vi "Passing Command Line Parameters.vi"() -> ()   [LabVIEW 2023]
doc: "This example shows how to use the Application:Command Line Arguments property to retrieve parameters that were returned when the LabVIEW executable was called from the command line.\n\nUse the following syntax in the Command Line to launch this VI:\n\n\"<full path to LabVIEW directory>\\labview.exe\" \"<full path to LabVIEW directory>\\examples\\Application Control\\VI Server\\Passing Command Line Parameters\\Command Line Target.vi\" This VI is set to run when opened.\n\nAfter the VI name, enter two hyphens (--) surrounded by spaces before the user-defined arguments. The arguments will be displayed in the front panel indicators. The correct syntax for arguments that can be passed is:\n\n/number:\n/boolean:\n/string:\nAfter (:) enter the appropriate value. If you enter more than one argument, they need to be separated with a space."
panel:
  out "Command Line String":string
  in  "String":string
  in  "Boolean":bool
  in  "Numeric":dbl
  # "Overview: Demonstrates how to call a VI, and pass parameters to the VI, through the command line.\nInstructions:\n1. Specify desired values for Numeric, Boolean and String.\n2. Run the VI.\n3. Highlight the text in the Command Line String indicator and select Edit > Copy to copy the text to the clipboard.\n4. Exit LabVIEW.\n5. Paste the string into a command line window and run the command. (To do this on Windows, press Window-R, type 'cmd', press Enter, right-click in the command window and select Paste, then press Enter.)"
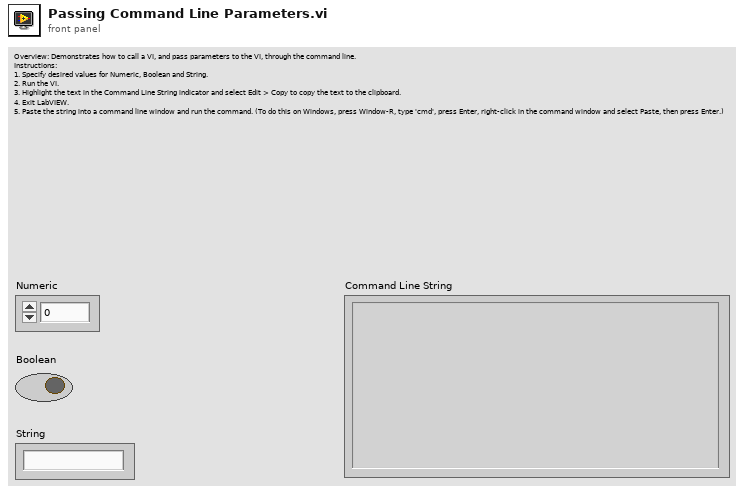
[diagram p1: front panel]
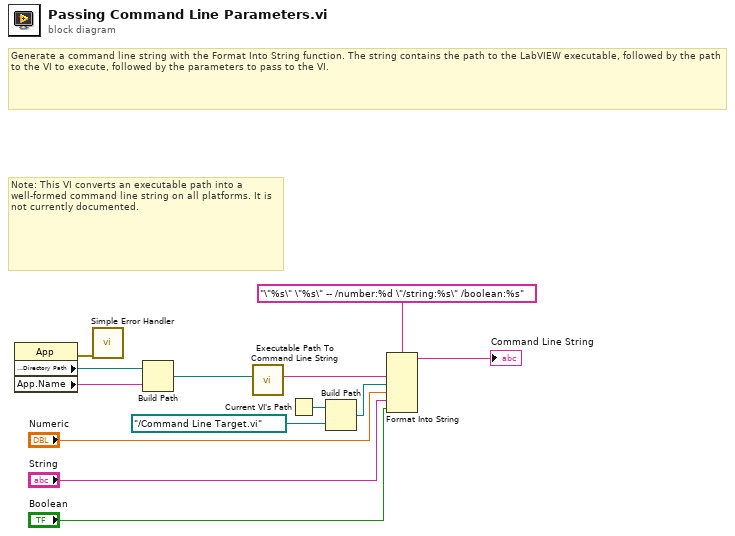
[diagram p0: block diagram]
diagram:
  # "Note: This VI converts an executable path into a well-formed command line string on all platforms. It is not currently documented."
  # "Generate a command line string with the Format Into String function. The string contains the path to the LabVIEW executable, followed by the path to the VI to execute, followed by the parameters to pass to the VI."
  n1 = property class="App"() -> (error out=w11:errorcluster, "Application:Directory Path"=w10:path, "App.Name"=w9:string)  [unwired: 2 in, 1 out]
  n2 = call <vilib>:"Simple Error Handler.vi"("error in (no error)"=w11) -> ()  [unwired: 1 in, 8 out]
  n3 = Build Path(base path=w10, name or relative path=w9) -> (appended path=w2:path)
  n4 = call <vilib>:"Executable Path To Command Line String.vi"("Executable Path"=w2) -> ("System Exec String"=w1:string)  [unwired: 10 in]
  n5 = Current VI's Path() -> (path=w13:path)
  n6 = Build Path(base path=w13, name or relative path=path "../Command Line Target.vi" ("path")) -> (appended path=w7:path)
  n7 = Format Into String(format string="\"%s\" \"%s\" -- /number:%d \"/string:%s\" /boolean:%s", w1, w7, "Numeric", "String", "Boolean") -> (resulting string=→"Command Line String":string)  [unwired: 2 in, 1 out]
